vi "calibrateSonar.vi"() -> ()   [LabVIEW 2014]
panel:
  out "Find starting position?":bool
  out "IR Distance Reading":dbl
  in  "stop":bool
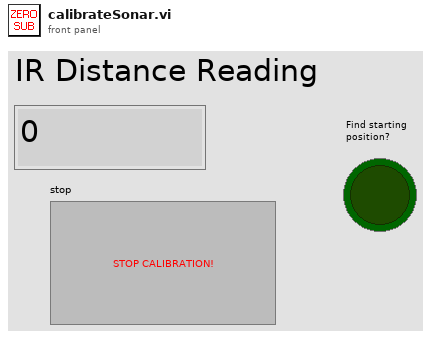
[diagram p1: front panel]
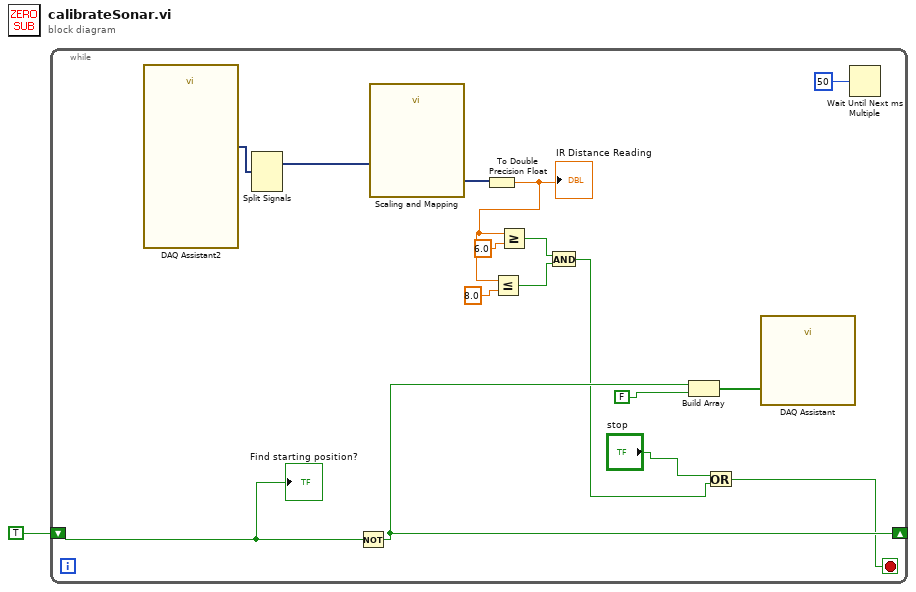
[diagram p0: block diagram]
diagram:
  n1 = while {
    shift-right: [w16] -> _
    shift-left: TRUE -> [w14]
    stop <- w4 stop-if-true
    n2 = call "DAQ Assistant2"() -> ("data"=w12:dynamicdata)  [unwired: 16 in, 3 out]
    n3 = Split Signals "Split Signals"(w12) -> (w13:dynamicdata)  [unwired: 5 in, 4 out]
    n4 = Not(x=w14) -> (.not. x?=w16:bool)
    n5 = call "Scaling and Mapping"("Signals"=w13) -> ("Scaled Signals"=w7:dynamicdata)  [unwired: 9 in, 1 out]
    n6 = To Double Precision Float(number=w7) -> (double precision float=w6:dbl)
    "IR Distance Reading" <- w6
    n7 = Less Or Equal?(x=w6, y=8.0) -> (x <= y?=w8:bool)
    n8 = Greater Or Equal?(x=w6, y=6.0) -> (x >= y?=w9:bool)
    n9 = And(x=w9, y=w8) -> (x .and. y?=w5:bool)
    n10 = Build Array(w16, FALSE) -> (w17:bool[])
    n11 = Or(x="stop", y=w5) -> (x .or. y?=w4:bool)
    n12 = call "DAQ Assistant"("data"=w17) -> ()  [unwired: 17 in, 2 out]
    n13 = Wait Until Next ms Multiple(millisecond multiple=50) -> ()  [unwired: 1 out]
    "Find starting position?" <- w14
  }
